vi "DETStatus-Com-Exec.vi"(8 "error in (no error)":errorcluster, 11 "Detector in":refnum<class "Detector.lvclass">) -> (0 "error out":errorcluster, 3 "Detector out":refnum<class "Detector.lvclass">)   [LabVIEW 2015, in "Detector.lvclass"]
uses:
  Detector.lvclass
  dependecies/ControlsVIs/Clusters-def/Message types.ctl
  dependecies/ControlsVIs/Clusters-def/Det-Reply-to-Connect-client.ctl
  dependecies/ControlsVIs/Clusters-def/SERVER-Commands.ctl
  Detector.lvclass/Detector.ctl
  GeneralFunctionality/GeneralFunctionality.lvclass/GeneralFunctionality.ctl
  Message/Message.lvclass
  Control/Control-Server/Control-Server.lvclass
  GeneralFunctionality/GeneralFunctionality.lvclass
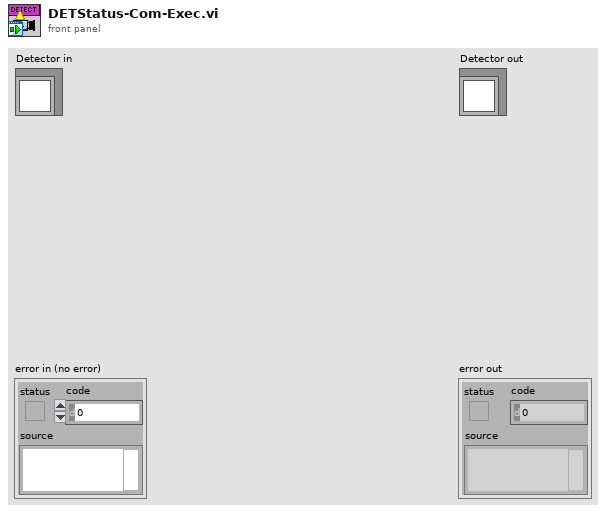
[diagram p1: front panel]
types:
  T1 = typedef "Control-Server.lvclass/SERVER-Commands.ctl" = string
  T2 = typedef "Detector.lvclass/Det-Reply-to-Connect-client.ctl" = cluster{"on/off":bool, "calibration":dbl[], "error":errorcluster}
  T3 = typedef "Message types.ctl" = string
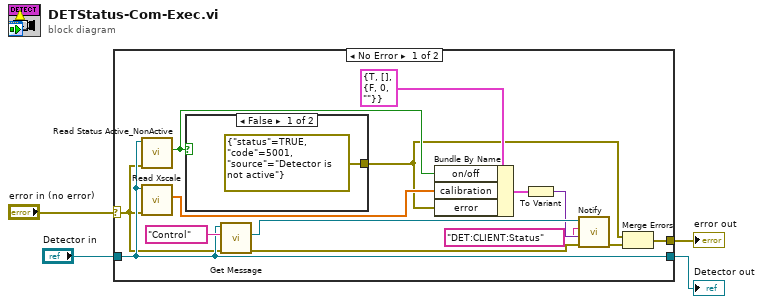
[diagram p0: block diagram]
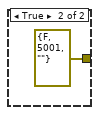
[diagram p2: hidden frame]
diagram:
  n1 = case shown="No Error" "error in (no error)" {
    selector: "error in (no error)" -> [w5 w22]
    tunnel: [w15 w22] -> w3
    tunnel: [w12 w21] -> w1
    tunnel: "Detector in" -> [w12 w21]
    frame No Error {
      n2 = call "Read Status Active_NonActive.vi"("error in (no error)"=w5, "GeneralFunctionality in"=w12) -> ("Status Active/NonActive"=w10:bool)  [unwired: 7 in, 2 out]
      n3 = call "Read Xscale.vi"("error in (no error)"=w5, "Detector en entrée"=w12) -> ("Xscale"=w11:dbl[])  [unwired: 7 in, 2 out]
      n4 = case shown="False" w10 {
        tunnel: [errorcluster {"status"=TRUE, "code"=5001, "source"="Detector is not active"} ("error") errorcluster {"status"=FALSE, "code"=5001, "source"=""} ("error")] -> w6
        frame False {
        }
        frame True {
        }
      }
      n5 = call "Get Message.vi"("error in (no error)"=w5, "Message type"=T3 "Control", "GeneralFunctionality en entrée"=w12) -> ("error out"=w14:errorcluster, "Message.lvclass"=w18:refnum<class "Message.lvclass">)  [unwired: 6 in, 1 out]
      n6 = Bundle By Name(cluster=T2 {"on/off"=TRUE, "calibration"=[], "error"={"status"=FALSE, "code"=0, "source"=""}}, "on/off"=w10, "calibration"=w11, "error"=w6) -> (w9:T2)
      n7 = To Variant(anything=w9) -> (Variant=w8:variant)
      n8 = call "Notify.vi"("error in (no error)"=w14, "Data"=w8, "command"=T1 "DET:CLIENT:Status" ("Commands"), "Message en entrée"=w18) -> ("error out"=w16:errorcluster)  [unwired: 6 in, 1 out]
      n9 = Merge Errors(w6, w16) -> (w15:errorcluster)
    }
    frame Error {
    }
  }
  "error out" <- w3
  "Detector out" <- w1
